vi "Backward Algorithm.vi"(10 "O Observed Sequence":i32[](array[numeric]), 11 "HMM Cluster":T1) -> (2 "Beta Partial Probalility":dbl[][](array[numeric]), 3 "Probability":dbl)   [LabVIEW 2014, in "HMM.lvlib"]
uses:
  HMM.lvlib
  Control/HMM Cluster.ctl
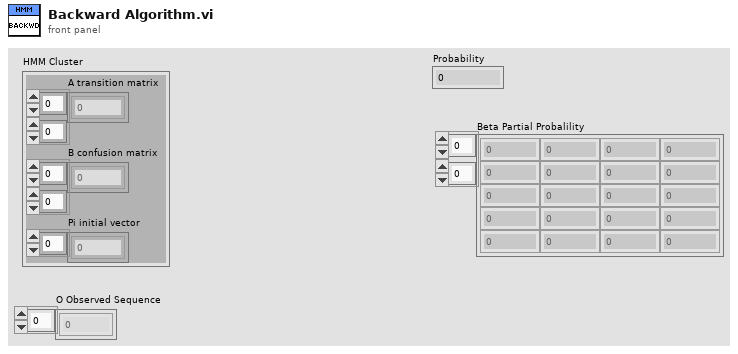
[diagram p1: front panel]
types:
  T1 = typedef "HMM.lvlib/HMM Cluster.ctl" = cluster{"A transition matrix":dbl[][], "B confusion matrix":dbl[][], "Pi initial vector":dbl[]}
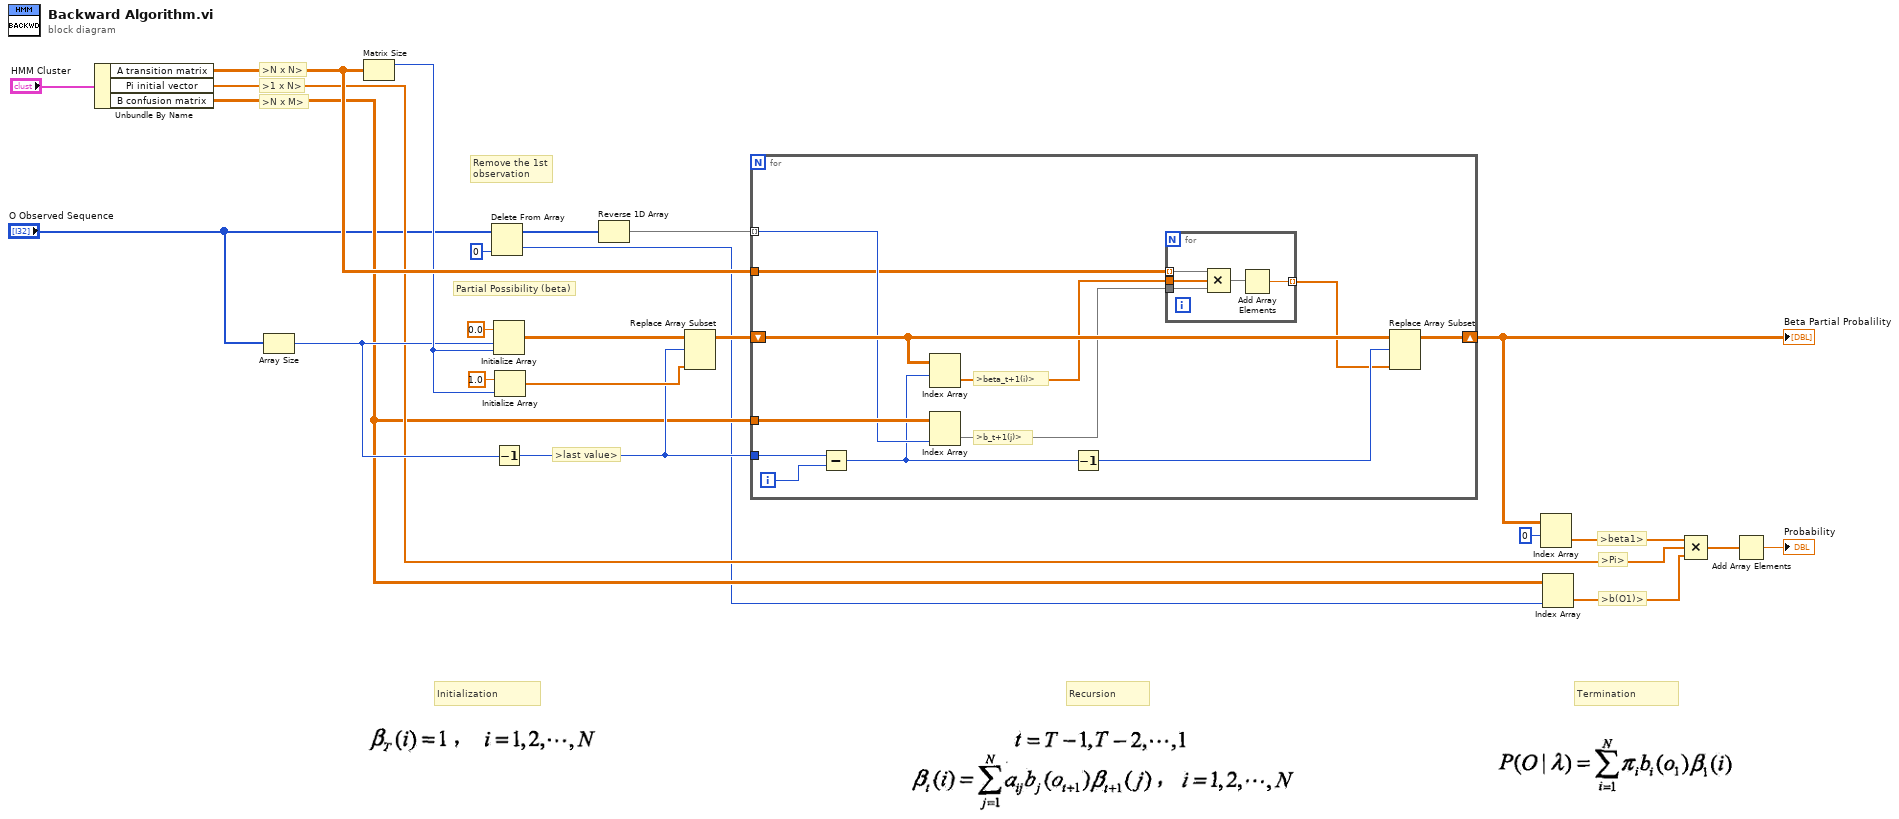
[diagram p0: block diagram]
diagram:
  # "Remove the 1st\nobservation"
  # ">beta1>"
  # ">b(O1)>"
  # ">Pi>"
  # ">last value>"
  # "Termination"
  # "Recursion"
  # "Initialization"
  # ">N x M>"
  # ">1 x N>"
  # ">N x N>"
  # "Partial Possibility (beta)"
  n1 = Unbundle By Name("HMM Cluster") -> ("A transition matrix"=w19:dbl[][], "Pi initial vector"=w9:dbl[], "B confusion matrix"=w8:dbl[][])
  n2 = Array Size(array="O Observed Sequence") -> (size(s)=w13:i32)
  n3 = Matrix Size(0:w19) -> (1:w15:i32)  [unwired: 1 out]
  n4 = Delete From Array(array="O Observed Sequence", index=0) -> (deleted portion=w2:i32, array with subset deleted=w4:i32[])  [unwired: 1 in]
  n5 = Initialize Array(0.0 ("element"), w13, w15) -> (w21:dbl[][])
  n6 = Decrement(x=w13) -> (x-1=w11:i32)
  n7 = Initialize Array(1.0 ("element"), w15) -> (w14:dbl[])
  n8 = Reverse 1D Array(array=w4) -> (reversed array=w12:i32[])
  n9 = Replace Array Subset(array=w21, new element=w14, index (row)=w11) -> (w20:dbl[][])  [unwired: 1 in]
  n10 = for {
    tunnel: w12 -> [w33] mode=indexing
    shift-right: [w29] -> w17
    shift-left: w20 -> [w35]
    tunnel: w19 -> [w27]
    tunnel: w8 -> [w34]
    tunnel: w11 -> [w32]
    i -> [w28]
    # ">beta_t+1(i)>"
    # ">b_t+1(j)>"
    n11 = Subtract(x=w32, y=w28) -> (x-y=w31:i32)
    n12 = Index Array(array=w35, index (row)=w31) -> (element=w26:dbl[])  [unwired: 1 in]
    n13 = Index Array(array=w34, index (col)=w33) -> (element=w25:dbl[])  [unwired: 1 in]
    n14 = Decrement(x=w31) -> (x-1=w30:i32)
    n15 = for {
      tunnel: w27 -> [w40] mode=indexing
      tunnel: w26 -> [w39]
      tunnel: w25 -> [w38]
      tunnel: [w36] -> w24 mode=indexing
      n16 = Compound Arithmetic op=MULTIPLY(w40, w39, w38) -> (w37:dbl[])
      n17 = Add Array Elements(numeric array=w37) -> (sum=w36:dbl)
    }
    n18 = Replace Array Subset(array=w35, new element=w24, index (row)=w30) -> (w29:dbl[][])  [unwired: 1 in]
  }
  "Beta Partial Probalility" <- w17
  n19 = Index Array(array=w17, index (row)=0) -> (element=w1:dbl[])  [unwired: 1 in]
  n20 = Index Array(array=w8, index (col)=w2) -> (element=w6:dbl[])  [unwired: 1 in]
  n21 = Compound Arithmetic op=MULTIPLY(w1, w9, w6) -> (w5:dbl[])
  n22 = Add Array Elements(numeric array=w5) -> (sum=→"Probability":dbl)
